vi "8164 Pset test.vi"() -> ()   [LabVIEW 2018]
uses:
  SPD Stand/typedefs/SPD.Stand Ctrl.ctl
  Instruments/SPD HID Interface/hidSPDLibForLabView/LibVIs/hidSPD Controls/hidSPD Device Session.ctl
  Instruments/SPD HID Interface/hidSPDLibForLabView/LibVIs/hidSPD Controls/hidSPD Controller.ctl
  Instruments/SPD HID Interface/hidSPDLibForLabView/LibVIs/hidSPD Controls/hidSPD SPD Type.ctl
  Instruments/KC705 DevBoard/typedefs/DevB.Session.ctl
  Instruments/KeySight 53230A/typedefs/FreqC.Session.ctl
  Instruments/KeySight 8164B/KeySight 8164B LAN InstrLib/typedefs/KeySight 8164B control.ctl
  Instruments/LeCroy SDA830/typedefs/LeCroy.Session.ctl
  SPD Stand/typedefs/SPD.Events.ctl
  SPD Stand/ConfigFile/SPD.Config File ctrl.ctl
  <vilib>/Utility/config.llb/Config Data RefNum.ctl
  SPD Stand/typedefs/SPD.Meas Result.ctl
  SPD Stand/typedefs/SPD.Queues.ctl
  SPD Stand/typedefs/SPD.Stand state.ctl
  Instruments/KeySight 8164B/KeySight 8164B LAN InstrLib.lvlib
  <vilib>/Utility/config.llb/NI_LVConfig.lvlib
  Instruments/SPD HID Interface/hidSPDLibForLabView/hidSPDLibForLabView.lvlib
panel:
  in  "Pset":dbl format="%#_6p"
  in  "stop":bool
  out "error out":errorcluster
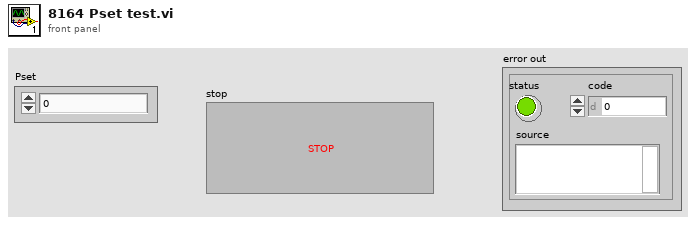
[diagram p1: front panel]
types:
  T1 = typedef "SPD.Stand Ctrl.ctl" = cluster{"spdDeviceSession":T2, "DevBSession":T5, "FreqCSession":T6, "8164BSession":T7, "LeCroySession":T8, "Events":T9, "configFile":T10, "SPD.Result":T12, "SPD.Queues":T13, "Console":refnum<vi>}
  T2 = typedef "hidSPDLibForLabView.lvlib/hidSPD Device Session.ctl" = cluster{"spdRef":u64, "connected":bool, "spdName":string, "hidSPD.Controller":T3, "hidSPD.Sturtup Values":T3, "SPD Type":T4}
  T3 = typedef "hidSPDLibForLabView.lvlib/hidSPD Controller.ctl" = cluster{"TSet":sgl, "HV_bias":sgl, "DDS_stb_code":u16}
  T4 = typedef "hidSPDLibForLabView.lvlib/hidSPD SPD Type.ctl" = enum16{"Free Run", "Gate"}
  T5 = typedef "DevB.Session.ctl" = cluster{"DevBRef":refnum<visa-resource-name>, "connected":bool}
  T6 = typedef "FreqC.Session.ctl" = cluster{"FreqCRef":refnum<visa-resource-name>, "timeout":dbl, "Gate":dbl, "connected":bool}
  T7 = typedef "KeySight 8164B LAN InstrLib.lvlib/KeySight 8164B control.ctl" = cluster{"Connection ID":refnum<k5>, "Connected":bool, "Info":string, "Slots Info":string[]}
  T8 = typedef "LeCroy.Session.ctl" = cluster{"LeCroySession":refnum<visa-resource-name>, "connected":bool}
  T9 = typedef "SPD.Events.ctl" = cluster{"DCRTest":refnum<user-event>, "Stop":refnum<user-event>}
  T10 = typedef "SPD.Config File ctrl.ctl" = cluster{"configFile ref":T11, "configFile path":path, "equipmentFile ref":T11}
  T11 = typedef "NI_LVConfig.lvlib/Config Data RefNum.ctl" = refnum<k1>
  T12 = typedef "SPD.Meas Result.ctl" = cluster{"HV_Bias":dbl[][][], "Stb_code":dbl[], "Temprature":dbl[], "Data":dbl[][][][], "DateTime":string}
  T13 = typedef "SPD.Queues.ctl" = cluster{"state queue":refnum<queue>}
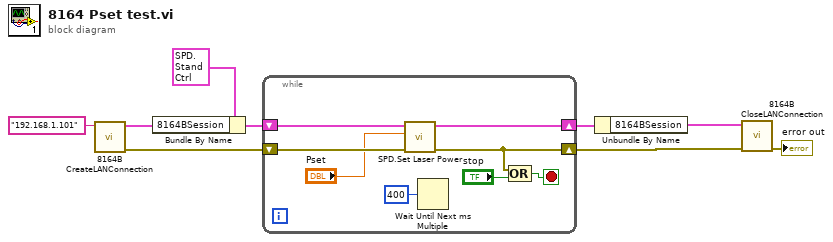
[diagram p0: block diagram]
diagram:
  n1 = call "8164B CreateLANConnection.vi"("IP address"="192.168.1.101") -> ("error out"=w5:errorcluster, "KeySight 8164B control out"=w6:T7)  [unwired: 9 in]
  n2 = Bundle By Name(cluster=T1 {"spdDeviceSession"={"spdRef"=0, "connected"=FALSE, "spdName"="", "hidSPD.Controller"={"TSet"=0.0, "HV_bias"=0.0, "DDS_stb_code"=0}, "hidSPD.Sturtup Values"={"TSet"=0.0, "HV_bias"=0.0, "DDS_stb_code"=0}, "SPD Type"=enum."Free Run"}, "DevBSession"={"DevBRef"="", "connected"=FALSE}, "FreqCSession"={"FreqCRef"="", "timeout"=0.0, "Gate"=0.0, "connected"=FALSE}, "8164BSession"={"Connection ID"=refnum, "Connected"=FALSE, "Info"="", "Slots Info"=[]}, "LeCroySession"={"LeCroySession"="", "connected"=FALSE}, "Events"={"DCRTest"=refnum, "Stop"=refnum}, "configFile"={"configFile ref"=refnum, "configFile path"=path "", "equipmentFile ref"=refnum}, "SPD.Result"={"HV_Bias"=[], "Stb_code"=[], "Temprature"=[], "Data"=[], "DateTime"=""}, "SPD.Queues"={"state queue"=refnum}, "Console"=refnum} ("SPD.Stand Ctrl in"), "8164BSession"=w6) -> (w4:T1)
  n3 = while {
    shift-right: [w10] -> w1
    shift-left: w5 -> [w17]
    shift-right: [w14] -> w3
    shift-left: w4 -> [w16]
    stop <- w12 stop-if-true
    n4 = call "SPD.Set Laser Power.vi"("Error In"=w17, "Pset"="Pset", "SPD.Stand Ctrl in"=w16) -> ("Error Out"=w10:errorcluster, "SPD.Stand Ctrl out"=w14:T1)  [unwired: 7 in]
    n5 = Wait Until Next ms Multiple(millisecond multiple=u32 400) -> ()  [unwired: 1 out]
    n6 = Compound Arithmetic op=OR(w10, "stop") -> (w12:bool)
  }
  n7 = Unbundle By Name(w3) -> ("8164BSession"=w2:T7)
  n8 = call "8164B CloseLANConnection.vi"("error in"=w1, "KeySight 8164B control"=w2) -> ("error out"=→"error out":errorcluster)  [unwired: 9 in]
